vi "Transient Response Conversion.vi"(0 "Trans Resp":T1 items=["Slow", "Normal", "Fast"]) -> (4 "Source:Transient Response":i32)   [LabVIEW 2024, in "devicePowerSequencerCoreLogic.lvlib"]
uses:
  devicePowerSequencerCoreLogic.lvlib
  controls/Transient Response.ctl
  Device Power Sequencer.lvlib
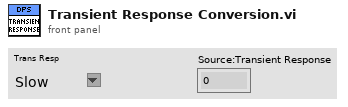
[diagram p1: front panel]
types:
  T1 = typedef "Device Power Sequencer.lvlib/Transient Response.ctl" = i32
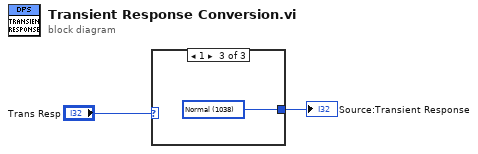
[diagram p0: block diagram]
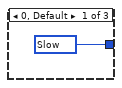
[diagram p2: hidden frame]
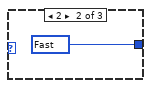
[diagram p3: hidden frame]
diagram:
  n1 = case shown="1" "Trans Resp" {
    tunnel: [w3 w4 w5] -> w1
    frame 0, Default {
      w3 = 1041 items=["Slow"=1041, "Normal"=1038, "Fast"=1039, "Custom"=1042] ("Source:Transient Response")
    }
    frame 2 {
      w4 = 1039 items=["Slow"=1041, "Normal"=1038, "Fast"=1039, "Custom"=1042] ("Source:Transient Response")
    }
    frame 1 {
      w5 = 1038 items=["Slow"=1041, "Normal"=1038, "Fast"=1039, "Custom"=1042] ("Source:Transient Response")
    }
  }
  "Source:Transient Response" <- w1
